vi "外观 1.vi"(0 "Data In":T5 caption="数据输入", 2 "Display State In":T3 caption="显示状态输入", 3 "Container State":T4 caption="容器状态") -> (6 "Data Out":T5 caption="数据输出", 7 "Display State Out":T3 caption="显示状态输出", 8 "Action":T2 caption="动作")   [LabVIEW 2016, in "曲线模型.xctl"]
uses:
  <vilib>/_xctls/Container State.ctl
  <vilib>/_xctls/Action.ctl
  <vilib>/_xctls/XControlSupport.lvlib
  <vilib>/Utility/config.llb/NI_LVConfig.lvlib
panel:
  in  "曲线模型":T1={"标液浓度1"=0.0, "样品1 F0"=0.0, "样品1 F1"=0.0, "测量吸光度1"=0.0, "样品1启用"=FALSE, "标液浓度2"=0.0, "样品2 F0"=0.0, "样品2 F1"=0.0, "测量吸光度2"=0.0, "样品2启用"=FALSE, "标液浓度3"=0.0, "样品3 F0"=0.0, "样品3 F1"=0.0, "测量吸光度3"=0.0, "样品3启用"=FALSE, "标液浓度4"=0.0, "样品4 F0"=0.0, "样品4 F1"=0.0, "测量吸光度4"=0.0, "样品4启用"=FALSE, "标液浓度5"=0.0, "样品5 F0"=0.0, "样品5 F1"=0.0, "测量吸光度5"=0.0, "样品5启用"=FALSE, "模型"=enum."线性", "method"=enum."最小二乘", "精度"=4.0, "XY图"=[], "拟合公式"="", "r^2"=0.0} {"r^2" format="%.7g"}
  # "标液浓度"
  # "F0"
  # "F1"
  # "吸光值显示"
  # "辅\n助\n计\n算\n区"
  # "样品一"
  # "样品二"
  # "样品三"
  # "样品四"
  # "样品五"
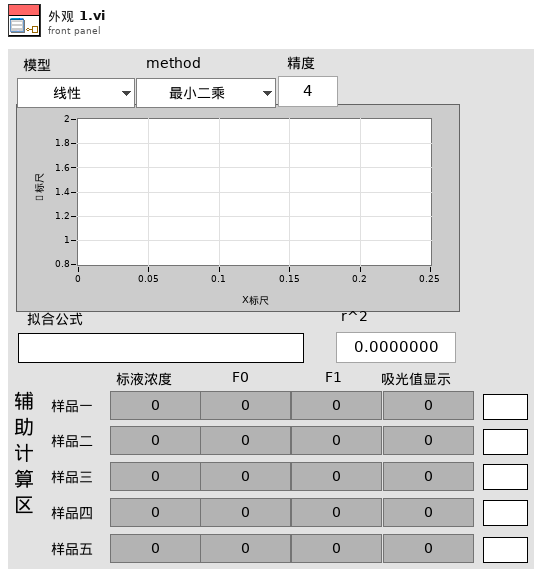
[diagram p1: front panel]
types:
  T1 = cluster{"标液浓度1":dbl, "样品1 F0":dbl, "样品1 F1":dbl, "测量吸光度1":dbl, "样品1启用":bool, "标液浓度2":dbl, "样品2 F0":dbl, "样品2 F1":dbl, "测量吸光度2":dbl, "样品2启用":bool, "标液浓度3":dbl, "样品3 F0":dbl, "样品3 F1":dbl, "测量吸光度3":dbl, "样品3启用":bool, "标液浓度4":dbl, "样品4 F0":dbl, "样品4 F1":dbl, "测量吸光度4":dbl, "样品4启用":bool, "标液浓度5":dbl, "样品5 F0":dbl, "样品5 F1":dbl, "测量吸光度5":dbl, "样品5启用":bool, "模型":enum32{"线性", "多项式"}, "method":enum16{"最小二乘", "最小绝对残差", "Bisquare"}, "精度":dbl, "XY图":cluster{"X Values":dbl[], "Y Values":dbl[]}[], "拟合公式":string, "r^2":dbl}
  T2 = typedef "XControlSupport.lvlib/Action.ctl" = cluster{"Data Changed?":bool, "State Changed?":bool, "Action Name":string}
  T3 = typedef "曲线模型.xctl/状态 1.ctl" = cluster{"模型选择":cluster{"参数":u8, "测量模式":u8, "量程":u8}, "吸光值":cluster{"Value":dbl, "Value 2":dbl, "Value 3":dbl, "Value 4":dbl, "Value 5":dbl}, "浓度":cluster{"标液浓度1":dbl, "标液浓度2":dbl, "标液浓度3":dbl, "标液浓度4":dbl, "标液浓度5":dbl}}
  T4 = typedef "XControlSupport.lvlib/Container State.ctl" = cluster{"Indicator?":bool, "Run Mode?":bool, " Refnum":refnum<vi>}
  T5 = typedef "曲线模型.xctl/数据 1.ctl" = cluster{"X^2":dbl, "X":dbl, "B":dbl}
  T6 = cluster{"曲线模型":cluster{"标液浓度1":dbl, "样品1 F0":dbl, "样品1 F1":dbl, "测量吸光度1":dbl, "样品1启用":bool, "标液浓度2":dbl, "样品2 F0":dbl, "样品2 F1":dbl, "测量吸光度2":dbl, "样品2启用":bool, "标液浓度3":dbl, "样品3 F0":dbl, "样品3 F1":dbl, "测量吸光度3":dbl, "样品3启用":bool, "标液浓度4":dbl, "样品4 F0":dbl, "样品4 F1":dbl, "测量吸光度4":dbl, "样品4启用":bool, "标液浓度5":dbl, "样品5 F0":dbl, "样品5 F1":dbl, "测量吸光度5":dbl, "样品5启用":bool, "模型":enum32{"线性", "多项式"}, "method":u16, "精度":dbl, "XY图":cluster{"X Values":dbl[], "Y Values":dbl[]}[], "拟合公式":string, "r^2":dbl}, "Polynomial Coefficients":dbl[]}
  T7 = cluster{"Value":dbl, "Value 2":dbl, "Value 3":dbl, "Value 4":dbl, "Value 5":dbl}
  T8 = typedef "NI_LVConfig.lvlib/Config Data RefNum.ctl" = refnum<k1>
  T9 = cluster{"Polynomial Coefficients[0]":dbl, "Polynomial Coefficients[1]":dbl, "Polynomial Coefficients[2]":dbl}
  T10 = cluster{"标液浓度1":dbl, "样品1 F0":dbl, "样品1 F1":dbl, "测量吸光度1":dbl, "样品1启用":bool, "标液浓度2":dbl, "样品2 F0":dbl, "样品2 F1":dbl, "测量吸光度2":dbl, "样品2启用":bool, "标液浓度3":dbl, "样品3 F0":dbl, "样品3 F1":dbl, "测量吸光度3":dbl, "样品3启用":bool, "标液浓度4":dbl, "样品4 F0":dbl, "样品4 F1":dbl, "测量吸光度4":dbl, "样品4启用":bool, "标液浓度5":dbl, "样品5 F0":dbl, "样品5 F1":dbl, "测量吸光度5":dbl, "样品5启用":bool, "模型":enum32{"线性", "多项式"}, "method":u16, "精度":dbl, "XY图":cluster{"X Values":dbl[], "Y Values":dbl[]}[], "拟合公式":string, "r^2":dbl}
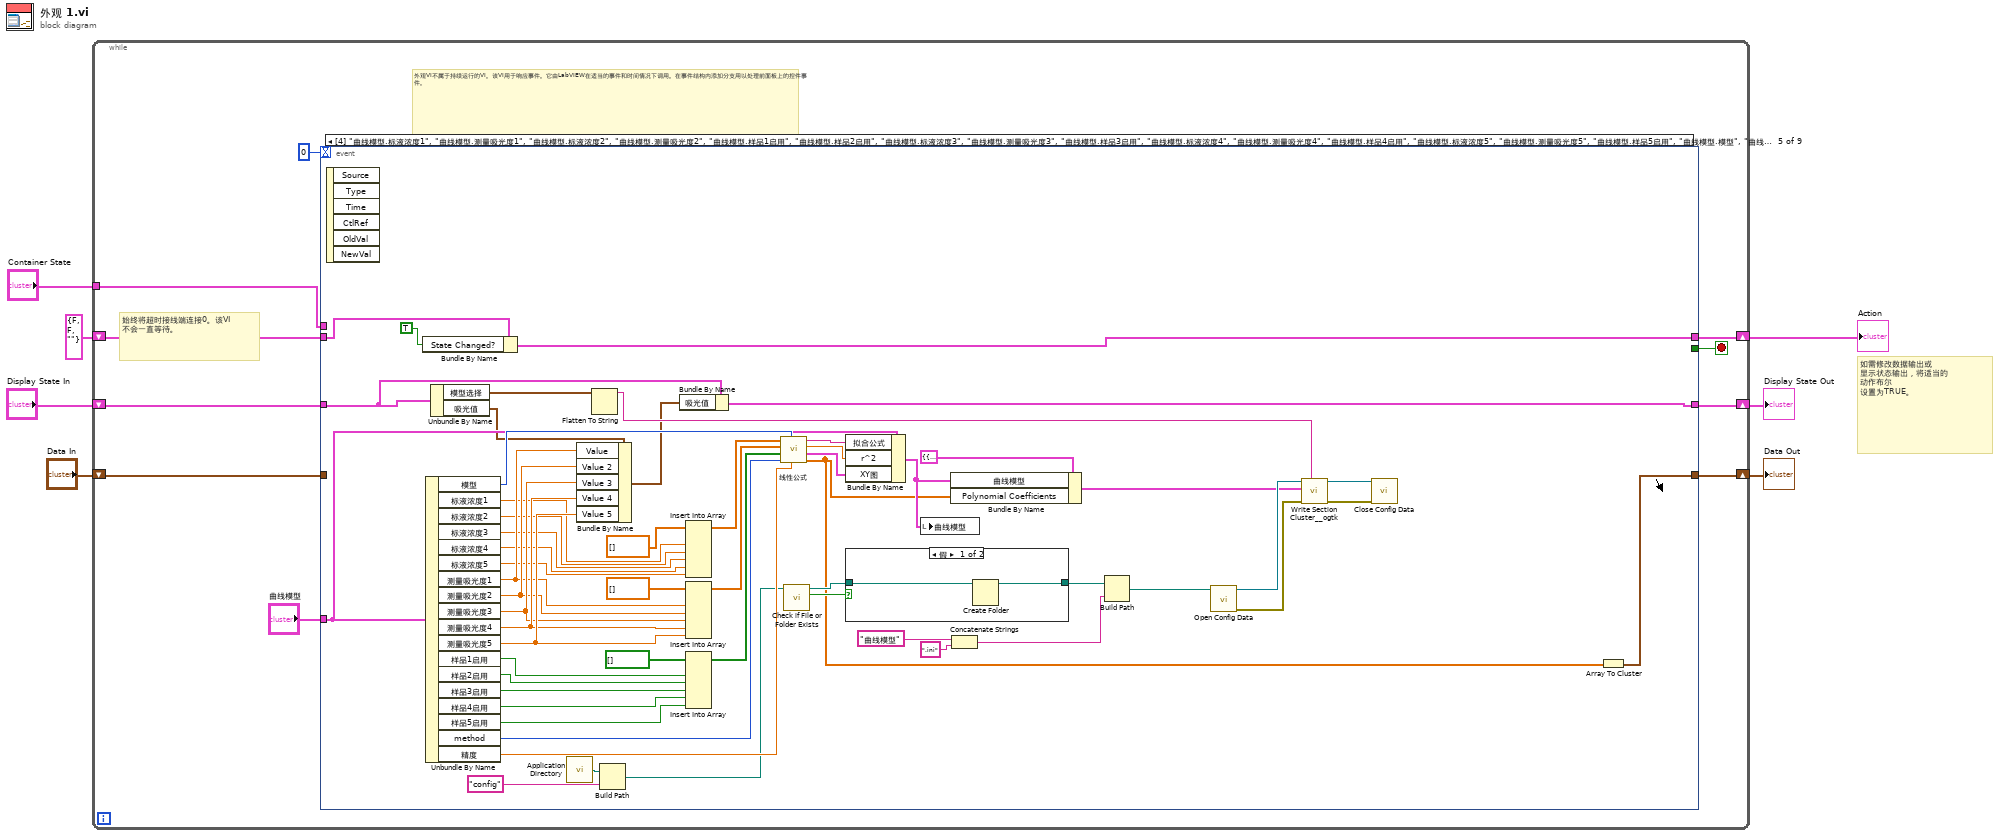
[diagram p0: block diagram]
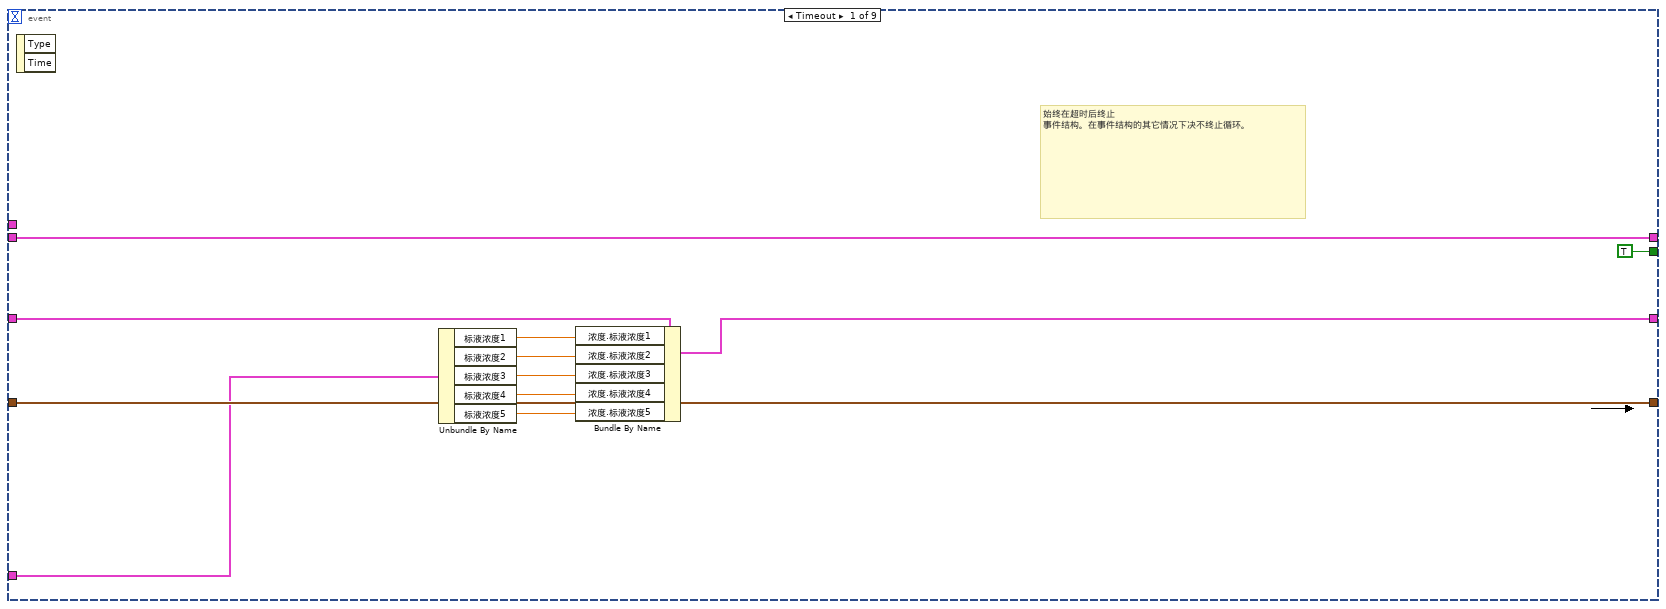
[diagram p2: hidden frame]
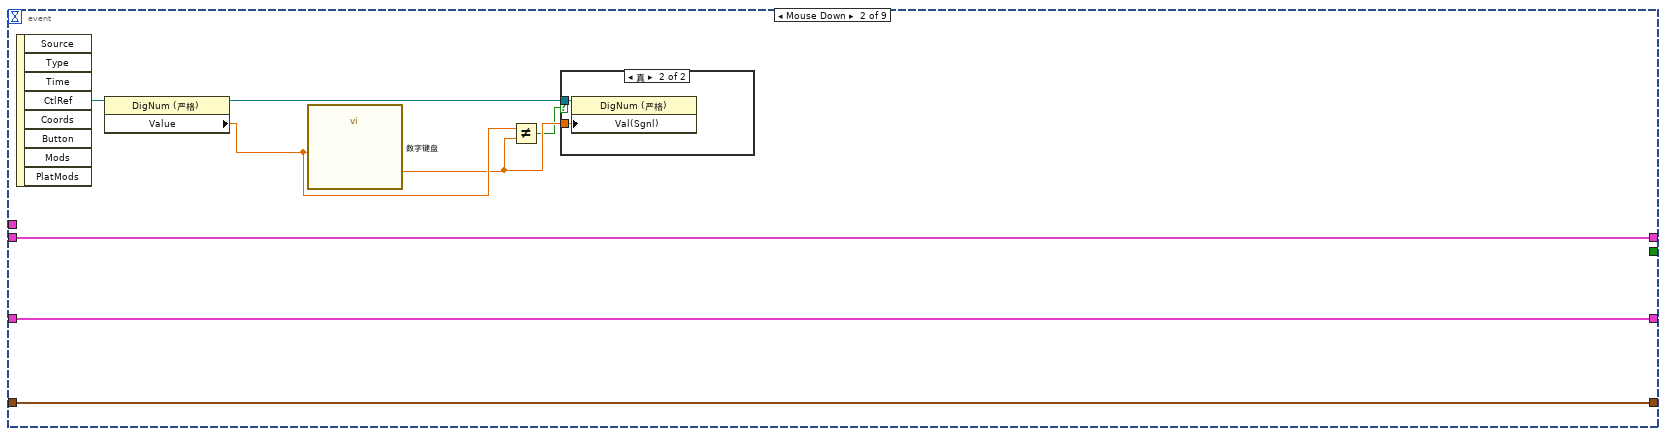
[diagram p3: hidden frame]
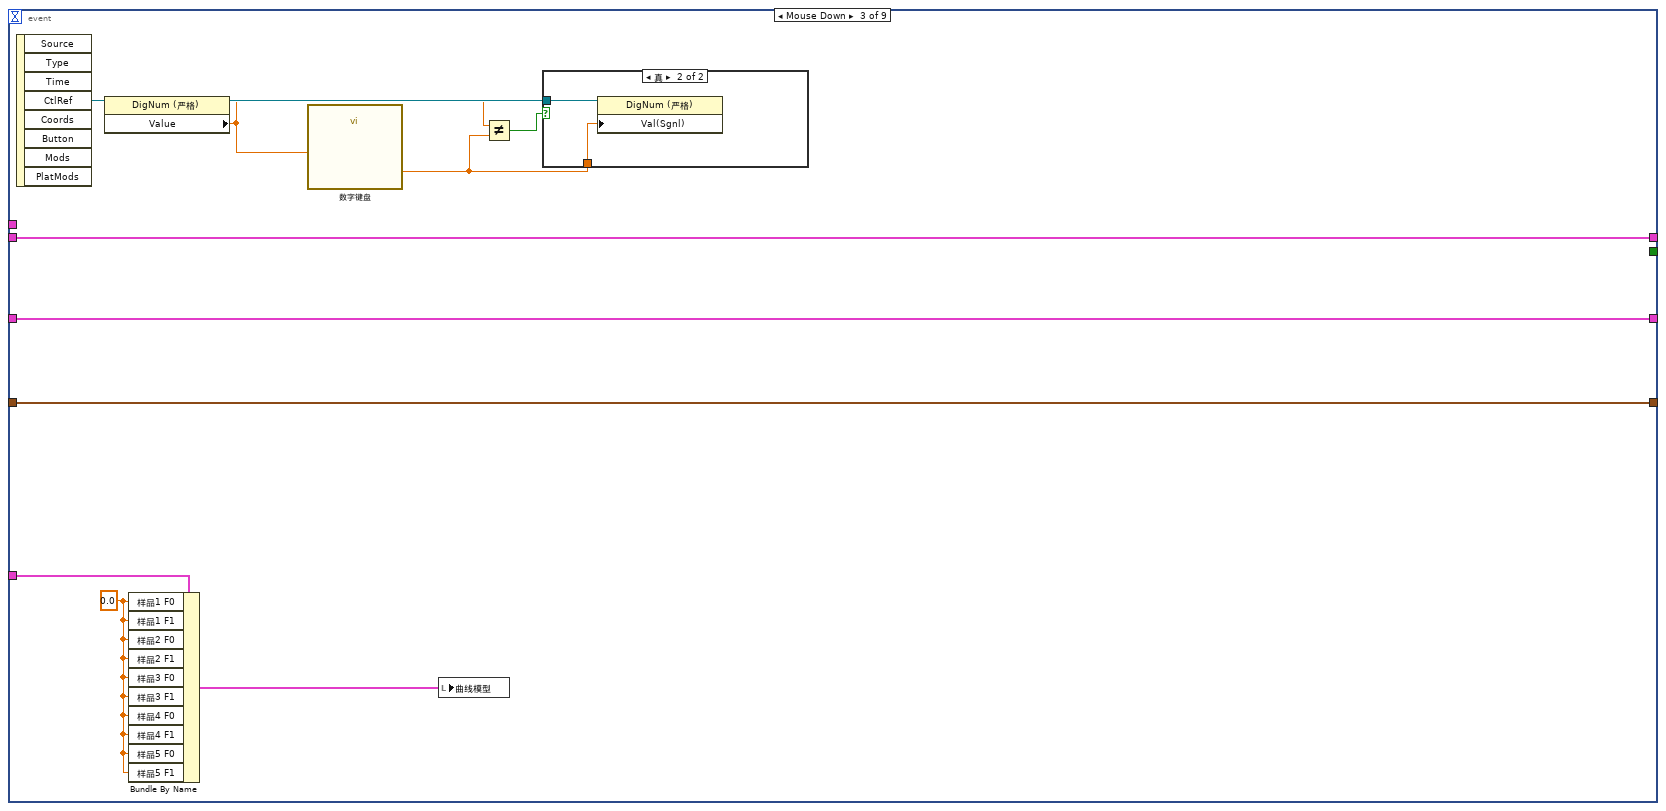
[diagram p5: hidden frame]
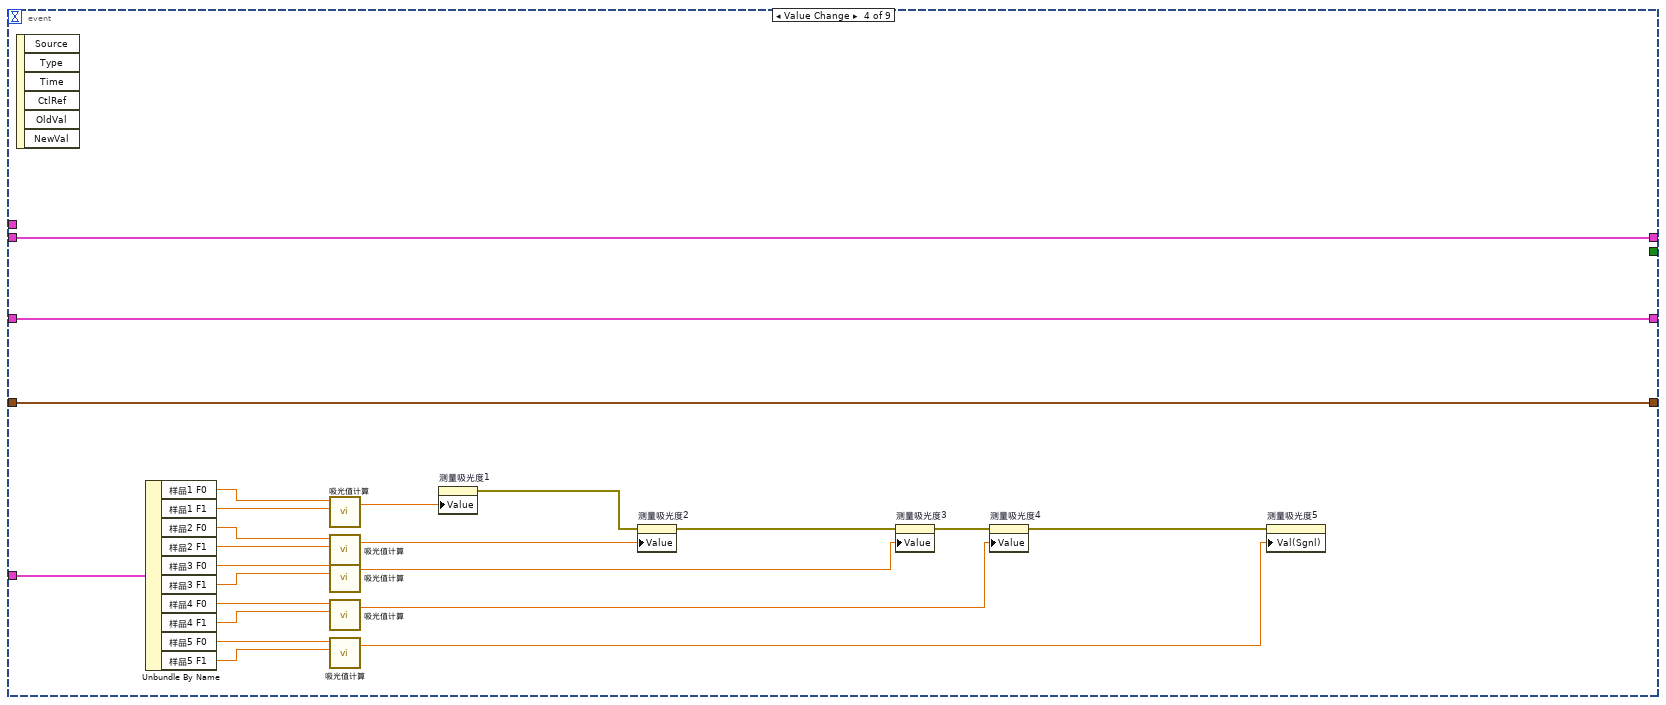
[diagram p7: hidden frame]
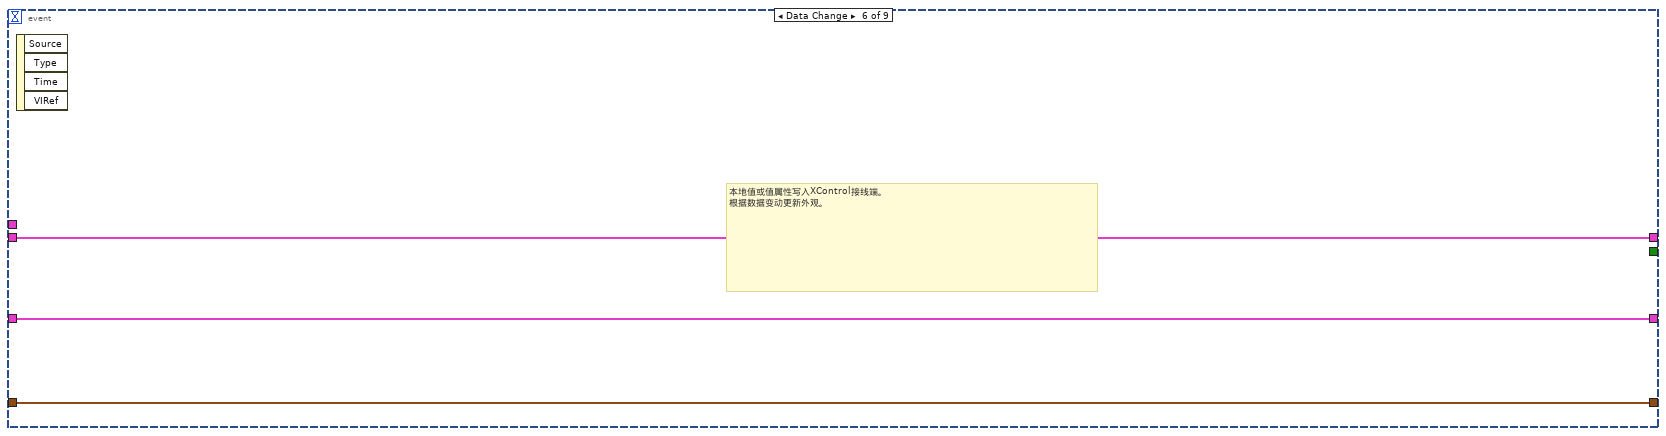
[diagram p9: hidden frame]
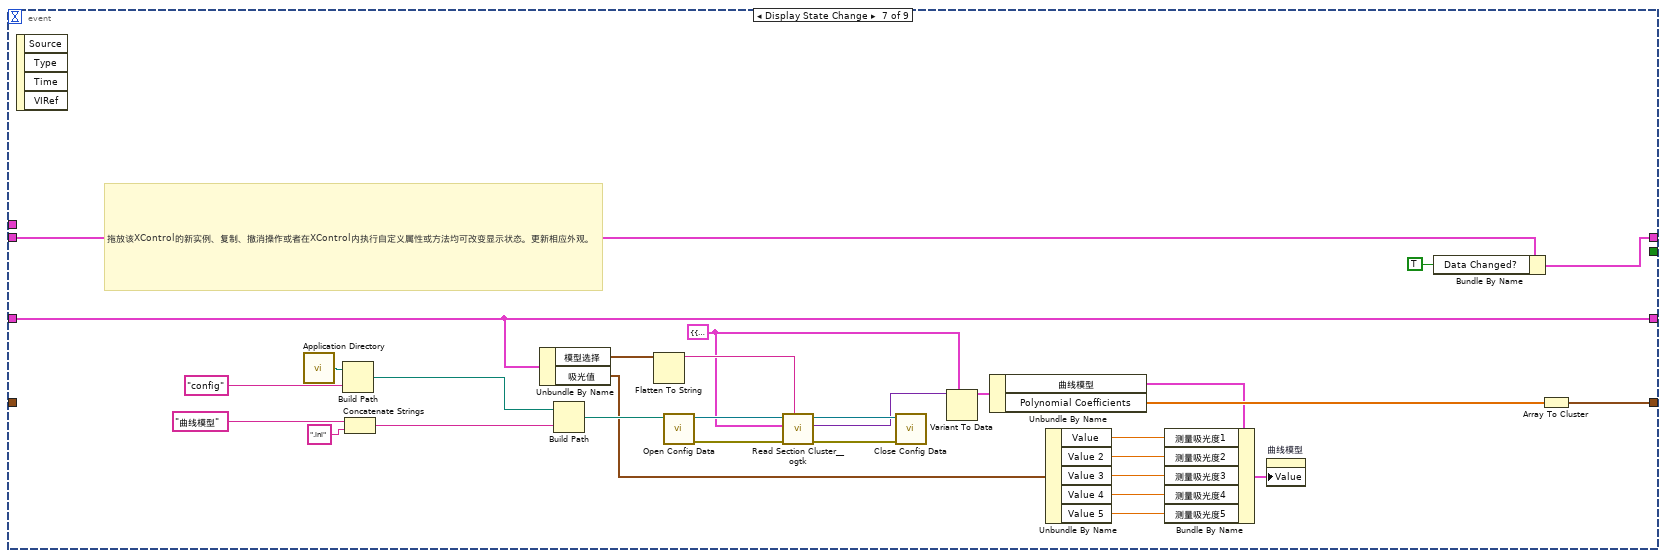
[diagram p10: hidden frame]
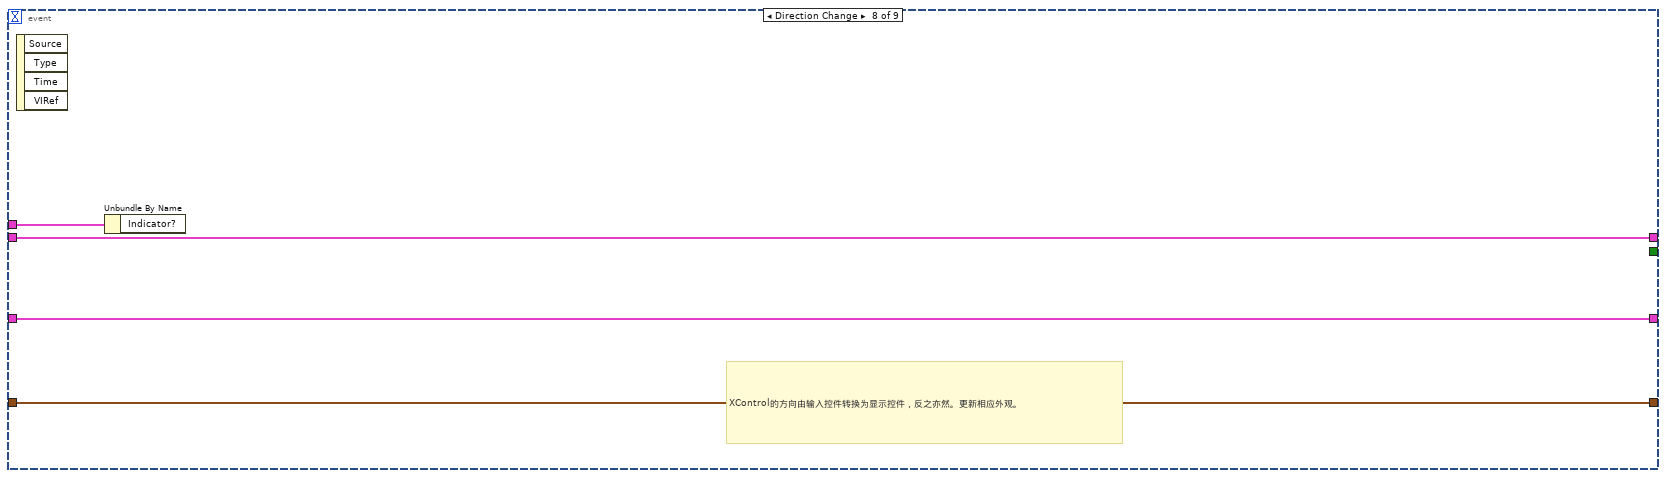
[diagram p11: hidden frame]
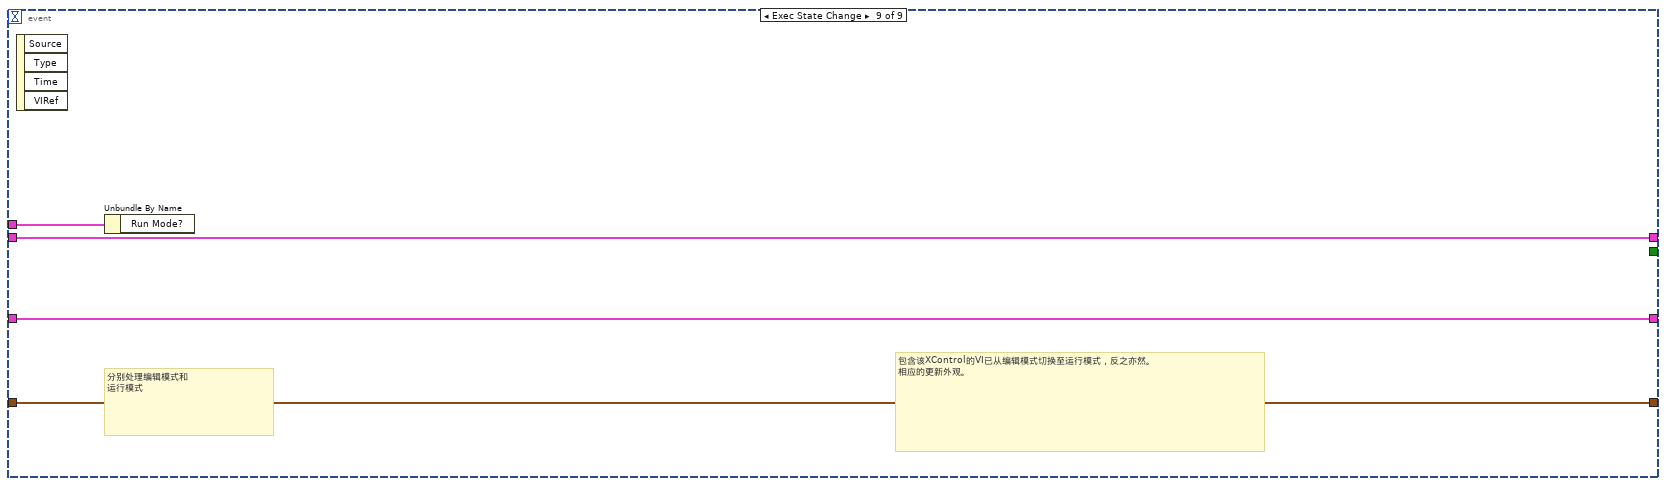
[diagram p12: hidden frame]
diagram:
  # "如需修改数据输出或\n显示状态输出，将适当的\n动作布尔\n设置为TRUE。"
  n1 = while {
    shift-right: [w16] -> w4
    shift-left: "Display State In" -> [w17]
    tunnel: "Container State" -> [w13]
    shift-right: [w11] -> w7
    shift-left: "Data In" -> [w12]
    shift-right: [w9] -> w2
    shift-left: T2 {"Data Changed?"=FALSE, "State Changed?"=FALSE, "Action Name"=""} ("Action") -> [w10]
    stop <- w15 stop-if-true
    # "外观VI不属于持续运行的VI。该VI用于响应事件。它由LabVIEW在适当的事件和时间情况下调用。在事件结构内添加分支用以处理前面板上的控件事件。"
    # "始终将超时接线端连接0。该VI\n不会一直等待。"
    n2 = event shown="[4] \"曲线模型.标液浓度1\", \"曲线模型.测量吸光度1\", \"曲线模型.标液浓度2\", \"曲线模型.测量吸光度2\", \"曲线模型.样品1启用\", \"曲线模型.样品2启用\", \"曲线模型.标液浓度3\", \"曲线模型.测量吸光度3\", \"曲线模型.样品3启用\", \"曲线模型.标液浓度4\", \"曲线模型.测量吸光度4\", \"曲线模型.样品4启用\", \"曲线模型.标液浓度5\", \"曲线模型.测量吸光度5\", \"曲线模型.样品5启用\", \"曲线模型.模型\", \"曲线模型.method\", \"曲线模型.精度\": 值改变" {
      selector: _ -> [_ _ _ _ _ _ _ _ _]
      dyn-events: _ -> [_ _ _ _ _ _ _ _ _]
      timeout: 0 -> [_ _ _ _ _ _ _ _ _]
      tunnel: w17 -> [w26 w32 w49 w74 w101 w134 w137 w169 w173]
      tunnel: [w24 w32 w49 w74 w88 w134 w137 w169 w173] -> w16
      tunnel: [TRUE _ _ _ _ _ _ _ _] -> w15
      tunnel: w13 -> [_ _ _ _ _ _ _ w170 w174]
      tunnel: w12 -> [w25 w36 w48 w73 _ w136 _ w168 w172]
      tunnel: [w25 w36 w48 w73 w112 w136 w149 w168 w172] -> w11
      tunnel: [w27 w35 w47 w72 w110 w135 w146 w167 w171] -> w9
      tunnel: w10 -> [w27 w35 w47 w72 w111 w135 w148 w167 w171]
      tunnel: "曲线模型" -> [w23 _ w44 w61 w116 _ _ _ _]
      event Timeout {
        # "始终在超时后终止\n事件结构。在事件结构的其它情况下决不终止循环。"
        n3 = event-data() -> ()  [unwired: 1 in, 2 out]
        n4 = Unbundle By Name(w23) -> ("标液浓度1"=w22:dbl, "标液浓度2"=w21:dbl, "标液浓度3"=w20:dbl, "标液浓度4"=w19:dbl, "标液浓度5"=w18:dbl)
        n5 = Bundle By Name(cluster=w26, "浓度.标液浓度1"=w22, "浓度.标液浓度2"=w21, "浓度.标液浓度3"=w20, "浓度.标液浓度4"=w19, "浓度.标液浓度5"=w18) -> (w24:T3)
      }
      event "曲线模型.标液浓度1", "曲线模型.样品1 F0", "曲线模型.样品1 F1", "曲线模型.标液浓度2", "曲线模型.样品2 F0", "曲线模型.样品2 F1", "曲线模型.标液浓度3", "曲线模型.样品3 F0", "曲线模型.样品3 F1", "曲线模型.标液浓度4", "曲线模型.样品4 F0", "曲线模型.样品4 F1", "曲线模型.标液浓度5", "曲线模型.样品5 F0", "曲线模型.样品5 F1", "曲线模型.精度": Mouse Down {
        n6 = event-data() -> ("CtlRef"=w34:refnum<vi>)  [unwired: 1 in, 7 out]
        n7 = property class="DigNum (严格)"(reference=w34) -> (reference out=w33:refnum<vi>, "Value"=w31:dbl)  [unwired: 1 in, 1 out]
        n8 = call "数字键盘.vi"("OldNumber"=w31) -> ("NewNumber"=w30:dbl)
        n9 = Not Equal?(x=w31, y=w30) -> (x != y?=w29:bool)
        n10 = case shown="真" w29 {
          tunnel: w33 -> [_ w38]
          tunnel: w30 -> [_ w37]
          frame False {
          }
          frame True {
            n11 = property class="DigNum (严格)"(reference=w38, "Val(Sgnl)"=w37) -> ()  [unwired: 1 in, 2 out]
          }
        }
      }
      event "曲线模型.测量吸光度1", "曲线模型.测量吸光度2", "曲线模型.测量吸光度3", "曲线模型.测量吸光度4", "曲线模型.测量吸光度5": Mouse Down {
        w43 = 0.0 ("测量吸光度1")
        n12 = event-data() -> ("CtlRef"=w46:refnum<vi>)  [unwired: 1 in, 7 out]
        n13 = property class="DigNum (严格)"(reference=w46) -> (reference out=w45:refnum<vi>, "Value"=w41:dbl)  [unwired: 1 in, 1 out]
        n14 = Bundle By Name(cluster=w44, "样品1 F0"=w43, "样品1 F1"=w43, "样品2 F0"=w43, "样品2 F1"=w43, "样品3 F0"=w43, "样品3 F1"=w43, "样品4 F0"=w43, "样品4 F1"=w43, "样品5 F0"=w43, "样品5 F1"=w43) -> (w42:T1)
        n15 = call "数字键盘.vi"("OldNumber"=w41) -> ("NewNumber"=w40:dbl)
        n16 = local write "曲线模型"(w42) -> ()
        n17 = Not Equal?(x=w41, y=w40) -> (x != y?=w39:bool)
        n18 = case shown="真" w39 {
          tunnel: w45 -> [_ w51]
          tunnel: w40 -> [_ w50]
          frame False {
          }
          frame True {
            n19 = property class="DigNum (严格)"(reference=w51, "Val(Sgnl)"=w50) -> ()  [unwired: 1 in, 2 out]
          }
        }
      }
      event "曲线模型.样品1 F0", "曲线模型.样品1 F1", "曲线模型.样品2 F0", "曲线模型.样品2 F1", "曲线模型.样品3 F0", "曲线模型.样品3 F1", "曲线模型.样品4 F0", "曲线模型.样品4 F1", "曲线模型.样品5 F0", "曲线模型.样品5 F1": Value Change {
        n20 = event-data() -> ()  [unwired: 1 in, 6 out]
        n21 = Unbundle By Name(w61) -> ("样品1 F0"=w71:dbl, "样品1 F1"=w70:dbl, "样品2 F0"=w62:dbl, "样品2 F1"=w63:dbl, "样品3 F0"=w64:dbl, "样品3 F1"=w65:dbl, "样品4 F0"=w66:dbl, "样品4 F1"=w67:dbl, "样品5 F0"=w68:dbl, "样品5 F1"=w69:dbl)
        n22 = call "吸光值计算.vi"("F1"=w70, "F0"=w71) -> ("测量吸光度"=w56:dbl)  [unwired: 3 in]
        n23 = call "吸光值计算.vi"("F1"=w63, "F0"=w62) -> ("测量吸光度"=w55:dbl)  [unwired: 3 in]
        n24 = call "吸光值计算.vi"("F1"=w65, "F0"=w64) -> ("测量吸光度"=w54:dbl)  [unwired: 3 in]
        n25 = call "吸光值计算.vi"("F1"=w67, "F0"=w66) -> ("测量吸光度"=w53:dbl)  [unwired: 3 in]
        n26 = call "吸光值计算.vi"("F1"=w69, "F0"=w68) -> ("测量吸光度"=w52:dbl)  [unwired: 3 in]
        n27 = property on="测量吸光度1" class="DigNum (严格)"("Value"=w56) -> (error out=w60:errorcluster)  [unwired: 2 in, 1 out]
        n28 = property on="测量吸光度2" class="DigNum (严格)"(error in=w60, "Value"=w55) -> (error out=w59:errorcluster)  [unwired: 1 in, 1 out]
        n29 = property on="测量吸光度3" class="DigNum (严格)"(error in=w59, "Value"=w54) -> (error out=w58:errorcluster)  [unwired: 1 in, 1 out]
        n30 = property on="测量吸光度4" class="DigNum (严格)"(error in=w58, "Value"=w53) -> (error out=w57:errorcluster)  [unwired: 1 in, 1 out]
        n31 = property on="测量吸光度5" class="DigNum (严格)"(error in=w57, "Val(Sgnl)"=w52) -> ()  [unwired: 1 in, 2 out]
      }
      event "曲线模型.标液浓度1", "曲线模型.测量吸光度1", "曲线模型.标液浓度2", "曲线模型.测量吸光度2", "曲线模型.样品1启用", "曲线模型.样品2启用", "曲线模型.标液浓度3", "曲线模型.测量吸光度3", "曲线模型.样品3启用", "曲线模型.标液浓度4", "曲线模型.测量吸光度4", "曲线模型.样品4启用", "曲线模型.标液浓度5", "曲线模型.测量吸光度5", "曲线模型.样品5启用", "曲线模型.模型", "曲线模型.method", "曲线模型.精度": Value Change {
        n32 = event-data() -> ()  [unwired: 1 in, 6 out]
        n33 = Bundle By Name(cluster=w111, "State Changed?"=TRUE ("Data Changed?")) -> (w110:T2)
        n34 = Unbundle By Name(w116) -> ("模型"=w130:enum32{"线性", "多项式"}, "标液浓度1"=w80:dbl, "标液浓度2"=w79:dbl, "标液浓度3"=w78:dbl, "标液浓度4"=w77:dbl, "标液浓度5"=w76:dbl, "测量吸光度1"=w81:dbl, "测量吸光度2"=w82:dbl, "测量吸光度3"=w83:dbl, "测量吸光度4"=w84:dbl, "测量吸光度5"=w85:dbl, "样品1启用"=w122:bool, "样品2启用"=w121:bool, "样品3启用"=w120:bool, "样品4启用"=w119:bool, "样品5启用"=w118:bool, "method"=w129:enum16{"最小二乘", "最小绝对残差", "Bisquare"}, "精度"=w128:dbl)
        n35 = Unbundle By Name(w101) -> ("模型选择"=w100:cluster{"参数":u8, "测量模式":u8, "量程":u8}, "吸光值"=w86:T7)
        n36 = call <vilib>:"Application Directory.vi"() -> ("Application Directory"=w109:path)
        n37 = Bundle By Name(cluster=w86, "Value"=w81, "Value 2"=w82, "Value 3"=w83, "Value 4"=w84, "Value 5"=w85) -> (w87:T7)
        n38 = Flatten To String(anything=w100) -> (data string=w99:string)  [unwired: 3 in, 2 out]
        n39 = Build Path(base path=w109, name or relative path="config" ("名称或相对路径")) -> (appended path=w107:path)
        n40 = Bundle By Name(cluster=w101, "吸光值"=w87) -> (w88:T3)
        n41 = Insert Into Array(array=dbl[] [] ("标液浓度"), new element #1=w80, new element #2=w79, new element #3=w78, new element #4=w77, new element #5=w76) -> (w126:dbl[])  [unwired: 1 in]
        n42 = Insert Into Array(array=dbl[] [] ("标液浓度"), new element #1=w81, new element #2=w82, new element #3=w83, new element #4=w84, new element #5=w85) -> (w124:dbl[])  [unwired: 1 in]
        n43 = Insert Into Array(array=bool[] [] ("启用"), new element #1=w122, new element #2=w121, new element #3=w120, new element #4=w119, new element #5=w118) -> (w117:bool[])  [unwired: 1 in]
        n44 = call "线性公式.vi"("精度"=w128, "模型"=w130, "method"=w129, "启用"=w117, "监测浓度"=w124, "标液浓度"=w126) -> ("Polynomial Coefficients"=w90:dbl[], "XY图"=w113:cluster{"X Values":dbl[], "Y Values":dbl[]}[], "r^2"=w114:dbl, "拟合方程"=w115:string)  [unwired: 2 in]
        n45 = call <vilib>:"Check if File or Folder Exists.vi"("path"=w107) -> ("file or folder exists?"=w106:bool, "dup path"=w105:path)  [unwired: 8 in, 1 out]
        n46 = Bundle By Name(cluster=w116, "拟合公式"=w115, "r^2"=w114, "XY图"=w113) -> (w91:T1)
        n47 = case shown="假" w106 {
          tunnel: w105 -> [w132 w133]
          tunnel: [w131 w133] -> w102
          frame False {
            n48 = Create Folder(path (use dialog)=w132) -> (created path=w131:path)  [unwired: 2 in, 2 out]
          }
          frame True {
          }
        }
        n49 = local write "曲线模型"(w91) -> ()
        n50 = Bundle By Name(cluster=T6 {"曲线模型"={"标液浓度1"=0.0, "样品1 F0"=0.0, "样品1 F1"=0.0, "测量吸光度1"=0.0, "样品1启用"=FALSE, "标液浓度2"=0.0, "样品2 F0"=0.0, "样品2 F1"=0.0, "测量吸光度2"=0.0, "样品2启用"=FALSE, "标液浓度3"=0.0, "样品3 F0"=0.0, "样品3 F1"=0.0, "测量吸光度3"=0.0, "样品3启用"=FALSE, "标液浓度4"=0.0, "样品4 F0"=0.0, "样品4 F1"=0.0, "测量吸光度4"=0.0, "样品4启用"=FALSE, "标液浓度5"=0.0, "样品5 F0"=0.0, "样品5 F1"=0.0, "测量吸光度5"=0.0, "样品5启用"=FALSE, "模型"=enum."线性", "method"=0, "精度"=4.0, "XY图"=[], "拟合公式"="", "r^2"=0.0}, "Polynomial Coefficients"=[]} ("输出簇"), "曲线模型"=w91, "Polynomial Coefficients"=w90) -> (w89:T6)
        n51 = Concatenate Strings("曲线模型" ("字符串"), ".ini" ("字符串")) -> (w104:string)
        n52 = Build Path(base path=w102, name or relative path=w104) -> (appended path=w93:path)
        n53 = call <vilib>:"Open Config Data.vi"("configuration file path"=w93) -> ("error out"=w96:errorcluster, "refnum"=w97:T8)  [unwired: 8 in, 1 out]
        n54 = call <userlib>:"Write Section Cluster__ogtk.vi"("section (optional)"=w99, "error in (no error)"=w96, "Section Formatted Cluster"=w89, "refnum"=w97) -> ("error out"=w94:errorcluster, "dup refnum"=w95:T8)  [unwired: 6 in]
        n55 = call <vilib>:"Close Config Data.vi"("error in (no error)"=w94, "refnum"=w95) -> ()  [unwired: 8 in, 2 out]
        n56 = Array To Cluster(array=w90) -> (cluster=w112:T9)
      }
      event Data Change {
        # "本地值或值属性写入XControl接线端。\n根据数据变动更新外观。"
        n57 = event-data() -> ()  [unwired: 1 in, 4 out]
      }
      event Display State Change {
        w152 = T6 {"曲线模型"={"标液浓度1"=0.0, "样品1 F0"=0.0, "样品1 F1"=0.0, "测量吸光度1"=0.0, "样品1启用"=FALSE, "标液浓度2"=0.0, "样品2 F0"=0.0, "样品2 F1"=0.0, "测量吸光度2"=0.0, "样品2启用"=FALSE, "标液浓度3"=0.0, "样品3 F0"=0.0, "样品3 F1"=0.0, "测量吸光度3"=0.0, "样品3启用"=FALSE, "标液浓度4"=0.0, "样品4 F0"=0.0, "样品4 F1"=0.0, "测量吸光度4"=0.0, "样品4启用"=FALSE, "标液浓度5"=0.0, "样品5 F0"=0.0, "样品5 F1"=0.0, "测量吸光度5"=0.0, "样品5启用"=FALSE, "模型"=enum."线性", "method"=0, "精度"=4.0, "XY图"=[], "拟合公式"="", "r^2"=0.0}, "Polynomial Coefficients"=[]} ("输出簇")
        # "拖放该XControl的新实例、复制、撤消操作或者在XControl内执行自定义属性或方法均可改变显示状态。更新相应外观。"
        n58 = event-data() -> ()  [unwired: 1 in, 4 out]
        n59 = call <vilib>:"Application Directory.vi"() -> ("Application Directory"=w161:path)
        n60 = Build Path(base path=w161, name or relative path="config" ("名称或相对路径")) -> (appended path=w159:path)
        n61 = Concatenate Strings("曲线模型" ("字符串"), ".ini" ("字符串")) -> (w157:string)
        n62 = Unbundle By Name(w137) -> ("模型选择"=w155:cluster{"参数":u8, "测量模式":u8, "量程":u8}, "吸光值"=w145:T7)
        n63 = Build Path(base path=w159, name or relative path=w157) -> (appended path=w162:path)
        n64 = Flatten To String(anything=w155) -> (data string=w154:string)  [unwired: 3 in, 2 out]
        n65 = call <vilib>:"Open Config Data.vi"("configuration file path"=w162) -> ("error out"=w165:errorcluster, "refnum"=w166:T8)  [unwired: 8 in, 1 out]
        n66 = call <userlib>:"Read Section Cluster__ogtk.vi"("section (optional)"=w154, "error in (no error)"=w165, "Section Formatted Cluster Type"=w152, "refnum"=w166) -> ("error out"=w163:errorcluster, "Section Formatted Cluster"=w156:variant, "dup refnum"=w164:T8)  [unwired: 3 in, 2 out]
        n67 = call <vilib>:"Close Config Data.vi"("error in (no error)"=w163, "refnum"=w164) -> ()  [unwired: 8 in, 2 out]
        n68 = Variant To Data(type=w152, Variant=w156) -> (data=w151:T6)  [unwired: 1 in, 1 out]
        n69 = Unbundle By Name(w151) -> ("曲线模型"=w138:T10, "Polynomial Coefficients"=w150:dbl[])
        n70 = Unbundle By Name(w145) -> ("Value"=w144:dbl, "Value 2"=w143:dbl, "Value 3"=w142:dbl, "Value 4"=w141:dbl, "Value 5"=w140:dbl)
        n71 = Bundle By Name(cluster=w138, "测量吸光度1"=w144, "测量吸光度2"=w143, "测量吸光度3"=w142, "测量吸光度4"=w141, "测量吸光度5"=w140) -> (w139:T10)
        n72 = property on="曲线模型" class="Clust (严格)"("Value"=w139) -> ()  [unwired: 2 in, 2 out]
        n73 = Bundle By Name(cluster=w148, "Data Changed?"=TRUE) -> (w146:T2)
        n74 = Array To Cluster(array=w150) -> (cluster=w149:T9)
      }
      event Direction Change {
        # "XControl的方向由输入控件转换为显示控件，反之亦然。更新相应外观。"
        n75 = event-data() -> ()  [unwired: 1 in, 4 out]
        n76 = Unbundle By Name(w170) -> ()  [unwired: 1 out]
      }
      event Exec State Change {
        # "包含该XControl的VI已从编辑模式切换至运行模式，反之亦然。\n相应的更新外观。"
        # "分别处理编辑模式和\n运行模式"
        n77 = event-data() -> ()  [unwired: 1 in, 4 out]
        n78 = Unbundle By Name(w174) -> ()  [unwired: 1 out]
      }
    }
  }
  "Display State Out" <- w4
  "Data Out" <- w7
  "Action" <- w2
